vi "Strip BOM.vi"(11 "String":string) -> (1 "BOM Found":bool, 2 "Encoding":T1, 3 "String without BOM":string)   [LabVIEW 2020, in "G-Unicode.lvlib"]
doc: "Strips the Byte Order Mark (BOM) from the text in <b>String</b>, if present. If a BOM is found the corresponding value in <b>Encoding</b> will be set, and <b>BOM Found</b> will be TRUE. If no BOM is found, <b>String without BOM</b> will be unchanged."
uses:
  G-Unicode.lvlib
  Controls/String Encoding.ctl
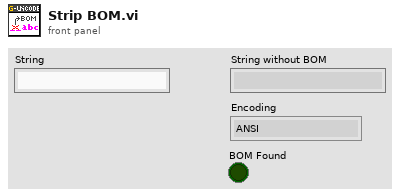
[diagram p1: front panel]
types:
  T1 = typedef "G-Unicode.lvlib/String Encoding.ctl" = enum16{"ANSI", "UTF-8", "UTF-16LE", "UTF-16BE", "Unknown"}
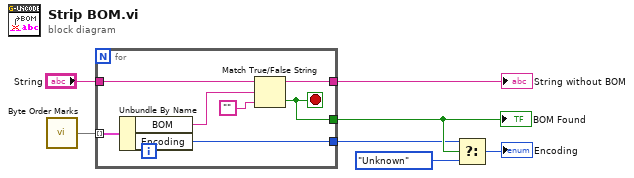
[diagram p0: block diagram]
diagram:
  n1 = call "Byte Order Marks.vi"() -> ("BOMs"=w1:map{T1, string})
  n2 = for {
    tunnel: "String" -> [w14]
    tunnel: [w13] -> w2
    tunnel: [w11] -> w6
    tunnel: [w8] -> w5
    tunnel: w1 -> [w10] mode=indexing
    stop <- w11 stop-if-true
    n3 = Unbundle By Name(w10) -> ("BOM"=w9:string, "Encoding"=w8:T1)
    n4 = Match True/False String(2:"", 3:w9, 4:w14) -> (0:w11:bool, 1:w13:string)
  }
  "BOM Found" <- w6
  "String without BOM" <- w2
  n5 = Select(t=w5, s=w6, f=String_Encoding."Unknown") -> (s? t:f=→"Encoding":T1)
